vi "Parallelizer Example.vi"   [LabVIEW 2017, in "Parallelizer Example.lvlib"]
uses:
  <vilib>/gpm_packages/@cs/test-executive/Source/Sandbox/Parallelizer Example/Parallelizer Example.lvlib
  <vilib>/gpm_packages/@cs/test-executive/Source/Test Executive/TestExecutive/Test Executive.lvclass
  C:/Program Files/National Instruments/LabVIEW 2017/vi.lib/gpm_packages/@cs/test-executive/Source/Test Executive/ITestExecutive/ITest Executive.lvclass
  <vilib>/gpm_packages/@cs/test-executive/Source/Sandbox/Parallelizer Example/Parallelizer/Parallelizer.lvclass
  <vilib>/gpm_packages/@cs/test-executive/Source/Sandbox/Parallelizer Example/Popup/Popup.lvclass
  <vilib>/gpm_packages/@cs/persistence/source/XML/XML.lvclass
  C:/Program Files/National Instruments/LabVIEW 2017/vi.lib/gpm_packages/@cs/persistence/source/IPersist/IPersist.lvclass
  <vilib>/gpm_packages/@cs/test-executive/Source/Sandbox/Parallelizer Example/Process Model/Process Model.lvclass
  C:/Program Files/National Instruments/LabVIEW 2017/vi.lib/ActorFramework/Actor/Actor.lvclass
  <vilib>/gpm_packages/@cs/test-executive/Source/Sandbox/Parallelizer Example/Process Model Messages/Create Process Msg/Create Process Msg.lvclass/Create Process Msg.ctl
  <vilib>/ActorFramework/Message Enqueuer/Message Enqueuer.lvclass/Message Enqueuer.ctl
  566084d9-bc61-4ed7-9f95-2e6a5a25145d.vi
  e2e0e614-b6b6-4dc5-81bb-3306618b8bec.vi
  64acf0f4-b7c5-4de8-beb0-ac56025c1a4d.vi
  951d23ca-1529-464f-8bdf-7408341acd11.vi
  20d732d3-35d4-4bdc-bbad-b8b414a28b1c.vi
  <vilib>/ActorFramework/Message Enqueuer/Enqueue.vi
  <vilib>/gpm_packages/@cs/test-executive/Source/Sandbox/Parallelizer Example/Process Model Messages/Create Process Msg/Create Process Msg.lvclass
  C:/Program Files/National Instruments/LabVIEW 2017/vi.lib/ActorFramework/Message/Message.lvclass
  <vilib>/Utility/error.llb/Error Cluster From Error Code.vi
  <vilib>/ActorFramework/Message Priority Queue/Priority Enqueue.vi
  <vilib>/gpm_packages/@cs/test-executive/Source/Test Executive/ITestExecutive/ITest Executive.lvclass
  <vilib>/gpm_packages/@cs/test-executive/Source/Test Executive/TestExecutive Ref/TestExecutive Ref.lvclass
  <vilib>/gpm_packages/@cs/test-executive/Source/Test Executive/Executioner/Executioner.lvclass
  <vilib>/ActorFramework/Actor/Actor.lvclass
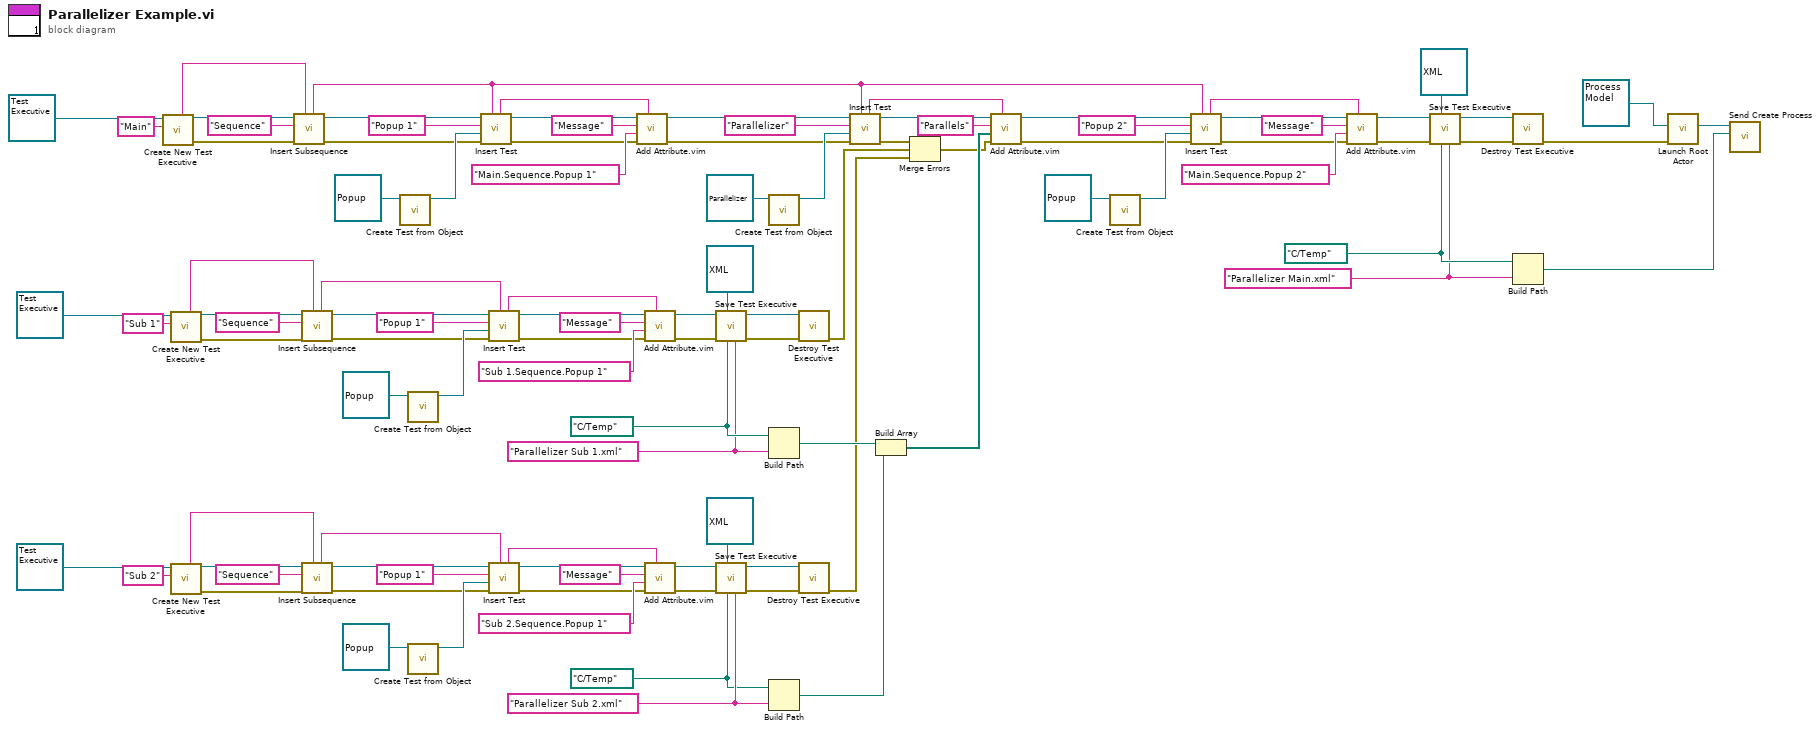
[diagram p0: block diagram]
diagram:
  w27 = "Parallelizer Sub 2.xml" ("File Name")
  w26 = path "C:/Temp" ("Folder")
  w28 = "Parallelizer Sub 1.xml" ("File Name")
  w29 = path "C:/Temp" ("Folder")
  w2 = "Parallelizer Main.xml" ("File Name")
  w3 = path "C:/Temp" ("Folder")
  n1 = call <vilib>:"Create New Test Executive.vi"("Name"="Main", "Test Executive"=refnum<class "Test Executive.lvclass"> refnum ("Test Executive.lvlib:Test Executive.lvclass")) -> ("error out"=w15:errorcluster, "Test Executive Ref"=w99:refnum<data-value>, "Test Executive ID out"=w98:string)  [unwired: 7 in]
  n2 = call <vilib>:"Create New Test Executive.vi"("Name"="Sub 1", "Test Executive"=refnum<class "Test Executive.lvclass"> refnum ("Test Executive.lvlib:Test Executive.lvclass")) -> ("error out"=w14:errorcluster, "Test Executive Ref"=w56:refnum<data-value>, "Test Executive ID out"=w57:string)  [unwired: 7 in]
  n3 = call <vilib>:"Create New Test Executive.vi"("Name"="Sub 2", "Test Executive"=refnum<class "Test Executive.lvclass"> refnum ("Test Executive.lvlib:Test Executive.lvclass")) -> ("error out"=w11:errorcluster, "Test Executive Ref"=w41:refnum<data-value>, "Test Executive ID out"=w40:string)  [unwired: 7 in]
  n4 = call <vilib>:"Insert Subsequence.vi"("Parent ID"=w98, "error in (no error)"=w15, "Name"="Sequence", "Test Executive Ref"=w99) -> ("error out"=w16:errorcluster, "Test Executive Ref out"=w96:refnum<data-value>, "Unique ID out"=w74:string)  [unwired: 4 in, 1 out]
  n5 = call <vilib>:"Insert Subsequence.vi"("Parent ID"=w57, "error in (no error)"=w14, "Name"="Sequence", "Test Executive Ref"=w56) -> ("error out"=w13:errorcluster, "Test Executive Ref out"=w59:refnum<data-value>, "Unique ID out"=w67:string)  [unwired: 4 in, 1 out]
  n6 = call <vilib>:"Insert Subsequence.vi"("Parent ID"=w40, "error in (no error)"=w11, "Name"="Sequence", "Test Executive Ref"=w41) -> ("error out"=w10:errorcluster, "Test Executive Ref out"=w38:refnum<data-value>, "Unique ID out"=w30:string)  [unwired: 4 in, 1 out]
  n7 = call <vilib>:"Create Test from Object.vi"("Test"=refnum<class "Popup.lvclass"> refnum ("Parallelizer Example.lvlib:Popup.lvclass")) -> ("Test"=w93:refnum<class "Executioner.lvclass">)  [unwired: 10 in]
  n8 = call <vilib>:"Create Test from Object.vi"("Test"=refnum<class "Popup.lvclass"> refnum ("Parallelizer Example.lvlib:Popup.lvclass")) -> ("Test"=w62:refnum<class "Executioner.lvclass">)  [unwired: 10 in]
  n9 = call <vilib>:"Create Test from Object.vi"("Test"=refnum<class "Popup.lvclass"> refnum ("Parallelizer Example.lvlib:Popup.lvclass")) -> ("Test"=w35:refnum<class "Executioner.lvclass">)  [unwired: 10 in]
  n10 = call <vilib>:"Insert Test.vi"("Parent ID"=w74, "error in (no error)"=w16, "Test"=w93, "Name"="Popup 1", "Test Executive Ref"=w96) -> ("error out"=w17:errorcluster, "Test Executive Ref out"=w92:refnum<data-value>, "Unique ID out"=w91:string)  [unwired: 3 in, 1 out]
  n11 = call <vilib>:"Insert Test.vi"("Parent ID"=w67, "error in (no error)"=w13, "Test"=w62, "Name"="Popup 1", "Test Executive Ref"=w59) -> ("error out"=w12:errorcluster, "Test Executive Ref out"=w63:refnum<data-value>, "Unique ID out"=w64:string)  [unwired: 3 in, 1 out]
  n12 = call <vilib>:"Insert Test.vi"("Parent ID"=w30, "error in (no error)"=w10, "Test"=w35, "Name"="Popup 1", "Test Executive Ref"=w38) -> ("error out"=w9:errorcluster, "Test Executive Ref out"=w34:refnum<data-value>, "Unique ID out"=w33:string)  [unwired: 3 in, 1 out]
  n13 = call "Add Attribute.vim"("ID"=w91, "error in (no error)"=w17, "Attribute"="Main.Sequence.Popup 1", "Attribute Name"="Message", "Test Executive Ref"=w92) -> ("error out"=w18:errorcluster, "Test Executive Ref out"=w86:refnum<data-value>)  [unwired: 3 in, 2 out]
  n14 = call "Add Attribute.vim"("ID"=w64, "error in (no error)"=w12, "Attribute"="Sub 1.Sequence.Popup 1", "Attribute Name"="Message", "Test Executive Ref"=w63) -> ("error out"=w49:errorcluster, "Test Executive Ref out"=w50:refnum<data-value>)  [unwired: 3 in, 2 out]
  n15 = call "Add Attribute.vim"("ID"=w33, "error in (no error)"=w9, "Attribute"="Sub 2.Sequence.Popup 1", "Attribute Name"="Message", "Test Executive Ref"=w34) -> ("error out"=w48:errorcluster, "Test Executive Ref out"=w47:refnum<data-value>)  [unwired: 3 in, 2 out]
  n16 = call <vilib>:"Save Test Executive.vi"("File Name"=w28, "Folder"=w29, "Persistence in"=refnum<class "XML.lvclass"> refnum ("XML.lvlib:XML.lvclass"), "error in (no error)"=w49, "Test Executive Ref"=w50) -> ("error out"=w53:errorcluster, "Test Executive Ref out"=w52:refnum<data-value>)  [unwired: 5 in]
  n17 = call <vilib>:"Save Test Executive.vi"("File Name"=w27, "Folder"=w26, "Persistence in"=refnum<class "XML.lvclass"> refnum ("XML.lvlib:XML.lvclass"), "error in (no error)"=w48, "Test Executive Ref"=w47) -> ("error out"=w44:errorcluster, "Test Executive Ref out"=w45:refnum<data-value>)  [unwired: 5 in]
  n18 = call <vilib>:"Create Test from Object.vi"("Test"=refnum<class "Parallelizer.lvclass"> refnum ("Parallelizer Example.lvlib:Parallelizer.lvclass")) -> ("Test"=w88:refnum<class "Executioner.lvclass">)  [unwired: 10 in]
  n19 = Build Path(base path=w29, name or relative path=w28) -> (appended path=w25:path)
  n20 = Build Path(base path=w26, name or relative path=w27) -> (appended path=w24:path)
  n21 = call <vilib>:"Destroy Test Executive.vi"("error in (no error)"=w53, "Test Executive Ref"=w52) -> ("error out"=w8:errorcluster)  [unwired: 9 in]
  n22 = call <vilib>:"Destroy Test Executive.vi"("error in (no error)"=w44, "Test Executive Ref"=w45) -> ("error out"=w7:errorcluster)  [unwired: 9 in]
  n23 = call <vilib>:"Insert Test.vi"("Parent ID"=w74, "error in (no error)"=w18, "Test"=w88, "Name"="Parallelizer", "Test Executive Ref"=w86) -> ("error out"=w20:errorcluster, "Test Executive Ref out"=w84:refnum<data-value>, "Unique ID out"=w83:string)  [unwired: 3 in, 1 out]
  n24 = Build Array(w25, w24) -> (w23:path[])
  n25 = Merge Errors(w20, w8, w7) -> (w19:errorcluster)
  n26 = call "Add Attribute.vim"("ID"=w83, "error in (no error)"=w19, "Attribute"=w23, "Attribute Name"="Parallels" ("Item Name"), "Test Executive Ref"=w84) -> ("error out"=w21:errorcluster, "Test Executive Ref out"=w75:refnum<data-value>)  [unwired: 3 in, 2 out]
  n27 = call <vilib>:"Create Test from Object.vi"("Test"=refnum<class "Popup.lvclass"> refnum ("Parallelizer Example.lvlib:Popup.lvclass")) -> ("Test"=w78:refnum<class "Executioner.lvclass">)  [unwired: 10 in]
  n28 = call <vilib>:"Insert Test.vi"("Parent ID"=w74, "error in (no error)"=w21, "Test"=w78, "Name"="Popup 2", "Test Executive Ref"=w75) -> ("error out"=w22:errorcluster, "Test Executive Ref out"=w79:refnum<data-value>, "Unique ID out"=w80:string)  [unwired: 3 in, 1 out]
  n29 = call "Add Attribute.vim"("ID"=w80, "error in (no error)"=w22, "Attribute"="Main.Sequence.Popup 2", "Attribute Name"="Message", "Test Executive Ref"=w79) -> ("error out"=w70:errorcluster, "Test Executive Ref out"=w71:refnum<data-value>)  [unwired: 3 in, 2 out]
  n30 = call <vilib>:"Save Test Executive.vi"("File Name"=w2, "Folder"=w3, "Persistence in"=refnum<class "XML.lvclass"> refnum ("XML.lvlib:XML.lvclass"), "error in (no error)"=w70, "Test Executive Ref"=w71) -> ("error out"=w68:errorcluster, "Test Executive Ref out"=w69:refnum<data-value>)  [unwired: 5 in]
  n31 = call <vilib>:"Destroy Test Executive.vi"("error in (no error)"=w68, "Test Executive Ref"=w69) -> ("error out"=w6:errorcluster)  [unwired: 9 in]
  n32 = Build Path(base path=w3, name or relative path=w2) -> (appended path=w1:path)
  n33 = call <vilib>:"Launch Root Actor.vi"("error in (no error)"=w6, "Actor"=refnum<class "Process Model.lvclass"> refnum ("Parallelizer Example.lvlib:Process Model.lvclass")) -> ("Actor's Enqueuer"=w4:refnum<class "Message Enqueuer.lvclass">)  [unwired: 8 in, 1 out]
  n34 = call <vilib>:"Send Create Process.vi"("Subroutine"=w1, "Message Enqueuer"=w4) -> ()  [unwired: 8 in, 2 out]
